vi "Config_Com_USB.vi"(0 "Enable":bool=TRUE, 2 "USB":T1={"COM"="", "baud rate (9600)"=9600, "data bits (8)"=8, "parity (0:none)"=enum."None", "stop bits (10: 1 bit)"=10, "flow control (0:none)"=0, "timeout (10sec)"=10000} {"stop bits (10: 1 bit)" items=["1.0"=10, "1.5"=15, "2.0"=20]; "flow control (0:none)" items=["None", "XON/XOFF", "RTS/CTS", "XON/XOFF & RTS/CTS", "DTR/DSR", "XON/XOFF & DTR/DSR"]}, 5 "error in (no error)":errorcluster) -> (17 "USB":T1={"COM"="", "baud rate (9600)"=9600, "data bits (8)"=8, "parity (0:none)"=enum."None", "stop bits (10: 1 bit)"=10, "flow control (0:none)"=0, "timeout (10sec)"=10000} {"stop bits (10: 1 bit)" items=["1.0"=10, "1.5"=15, "2.0"=20]; "flow control (0:none)" items=["None", "XON/XOFF", "RTS/CTS", "XON/XOFF & RTS/CTS", "DTR/DSR", "XON/XOFF & DTR/DSR"]}, 18 "OK":bool, 19 "error out":errorcluster)   [LabVIEW 2016]
doc: "Displays a standard dialog box that prompts users to enter information, such as a user name and password.\n--------------------\n\nThis Express VI is configured as follows:\n\nMessage to Display to the User:\nThe inputs are: \nNumber: sdfsdf"
panel:
  in  "COM USB CONFIG":T1={"COM"="", "baud rate (9600)"=9600, "data bits (8)"=8, "parity (0:none)"=enum."None", "stop bits (10: 1 bit)"=10, "flow control (0:none)"=0, "timeout (10sec)"=10000} {"stop bits (10: 1 bit)" items=["1.0"=10, "1.5"=15, "2.0"=20]; "flow control (0:none)" items=["None", "XON/XOFF", "RTS/CTS", "XON/XOFF & RTS/CTS", "DTR/DSR", "XON/XOFF & DTR/DSR"]}
  out "String":string
  in  "Cancel":bool
  in  "OK2":bool
  in  "OK1":bool
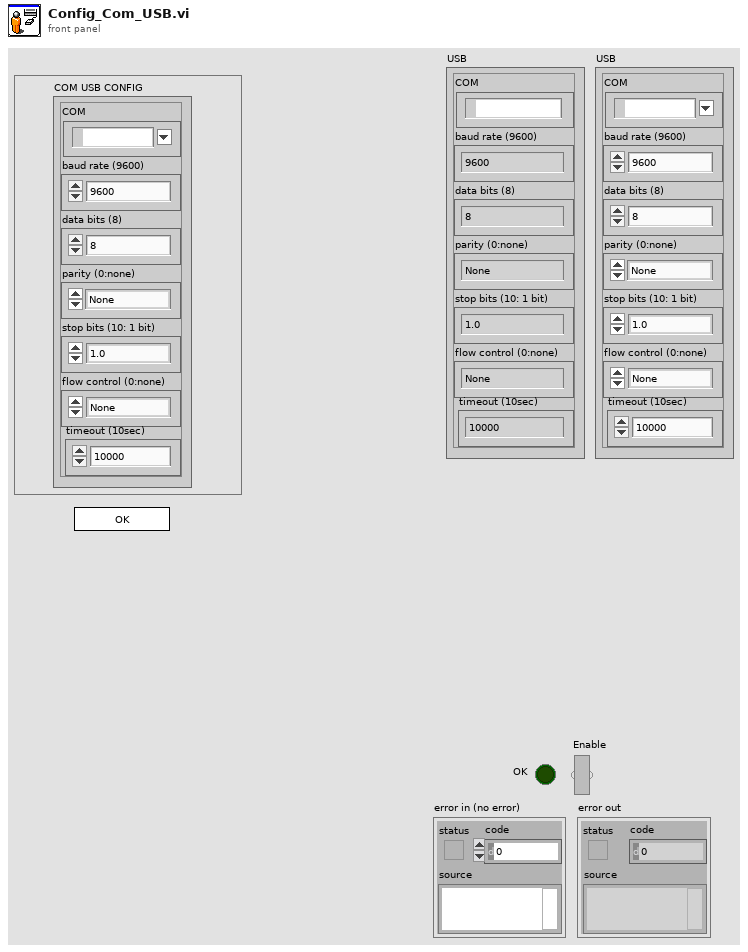
[diagram p1: front panel]
types:
  T1 = cluster{"COM":refnum<visa-resource-name>, "baud rate (9600)":u32, "data bits (8)":u16, "parity (0:none)":enum16{"None", "Odd", "Even", "Mark", "Space"}, "stop bits (10: 1 bit)":u16, "flow control (0:none)":u16, "timeout (10sec)":u32}
  T2 = cluster{"Input Name":string, "Input Data Type":i32}[]
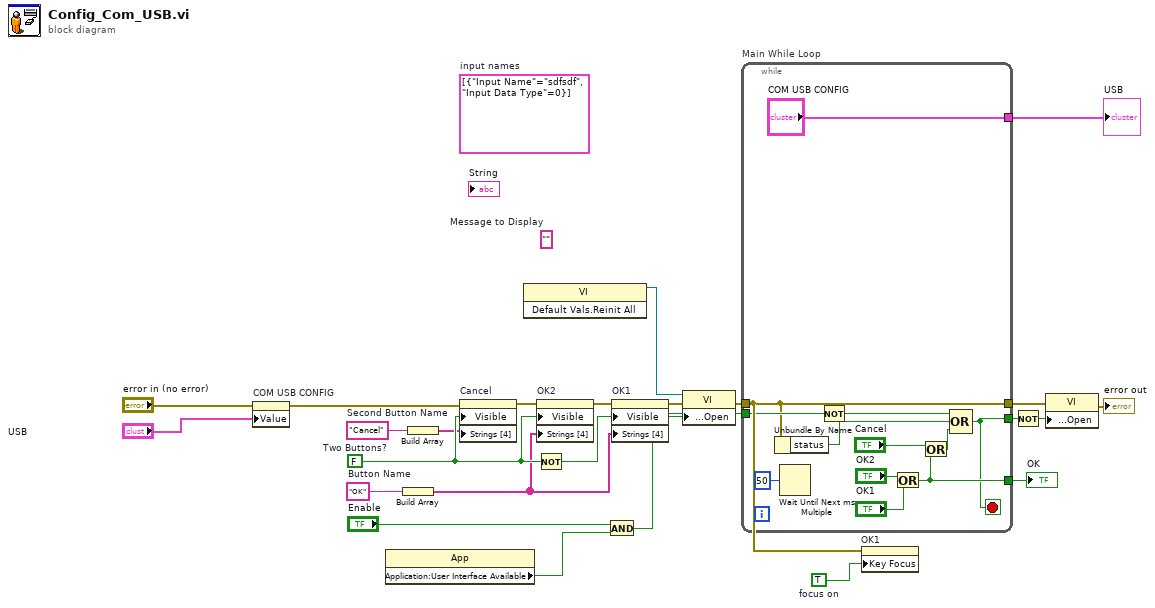
[diagram p0: block diagram]
diagram:
  w4 = TRUE  # focus on
  (unwired) T2 [{"Input Name"="sdfsdf", "Input Data Type"=0}]  # input names
  w16 = "Cancel"  # Second Button Name
  w14 = "OK"  # Button Name
  (unwired) ""  # Message to Display
  w24 = FALSE  # Two Buttons?
  n1 = property on="COM USB CONFIG" class="Clust (strict)"(error in="error in (no error)", "Value"="USB") -> (error out=w2:errorcluster)  [unwired: 1 in, 1 out]
  n2 = property class="App"() -> ("Application:User Interface Available"=w8:bool)  [unwired: 2 in, 2 out]
  n3 = Build Array(w14) -> (w15:string[])
  n4 = Build Array(w16) -> (w17:string[])
  n5 = property on="Cancel" class="Bool"(error in=w2, "Visible"=w24, "Strings [4]"=w17) -> (error out=w21:errorcluster)  [unwired: 1 in, 1 out]
  n6 = invoke class="VI" method="Default Vals.Reinit All"() -> (reference out=w7:refnum<vi>)  [unwired: 3 in, 2 out]
  n7 = Not(x=w24) -> (.not. x?=w22:bool)
  n8 = property on="OK2" class="Bool"(error in=w21, "Visible"=w24, "Strings [4]"=w15) -> (error out=w20:errorcluster)  [unwired: 1 in, 1 out]
  n9 = And(x="Enable", y=w8) -> (x .and. y?=w9:bool)
  n10 = property on="OK1" class="Bool"(error in=w20, "Visible"=w22, "Strings [4]"=w15) -> (error out=w13:errorcluster)  [unwired: 1 in, 1 out]
  n11 = property class="VI"(reference=w7, error in=w13, "Front Panel Window:Open"=w9) -> (error out=w5:errorcluster)  [unwired: 1 out]
  n12 = while "Main While Loop" {
    tunnel: [w33] -> w23
    tunnel: w9 -> [w31]
    tunnel: [w29] -> w18
    tunnel: w5 -> [w28]
    tunnel: [w28] -> w12
    tunnel: ["COM USB CONFIG"] -> w6
    stop <- w29 stop-if-true
    n13 = Unbundle By Name(w28) -> ("status"=w26:bool)
    n14 = Wait Until Next ms Multiple(millisecond multiple=u32 50) -> ()  [unwired: 1 out]
    n15 = Not(x=w31) -> (.not. x?=w30:bool)
    n16 = Or(x="OK2", y="OK1") -> (x .or. y?=w33:bool)
    n17 = Or(x="Cancel", y=w33) -> (x .or. y?=w27:bool)
    n18 = Compound Arithmetic op=OR(w30, w26, w27) -> (w29:bool)
  }
  "OK" <- w23
  "USB" <- w6
  n19 = property on="OK1" class="Bool"(error in=w5, "Key Focus"=w4) -> ()  [unwired: 1 in, 2 out]
  n20 = Not(x=w18) -> (.not. x?=w19:bool)
  n21 = property class="VI"(error in=w12, "Front Panel Window:Open"=w19) -> (error out=→"error out":errorcluster)  [unwired: 1 in, 1 out]
